vi "PC_Shot_Calculations (DONE).vi"(5 "Table Walls Input":sgl[](array[numeric]), 7 "Player and Puck Input":T1, 8 "Error In":errorcluster) -> (0 "Error Out":errorcluster, 2 "Shot Outputs":cluster{"Bounce":dbl[][], "Straight":dbl[][]})   [LabVIEW 2017]
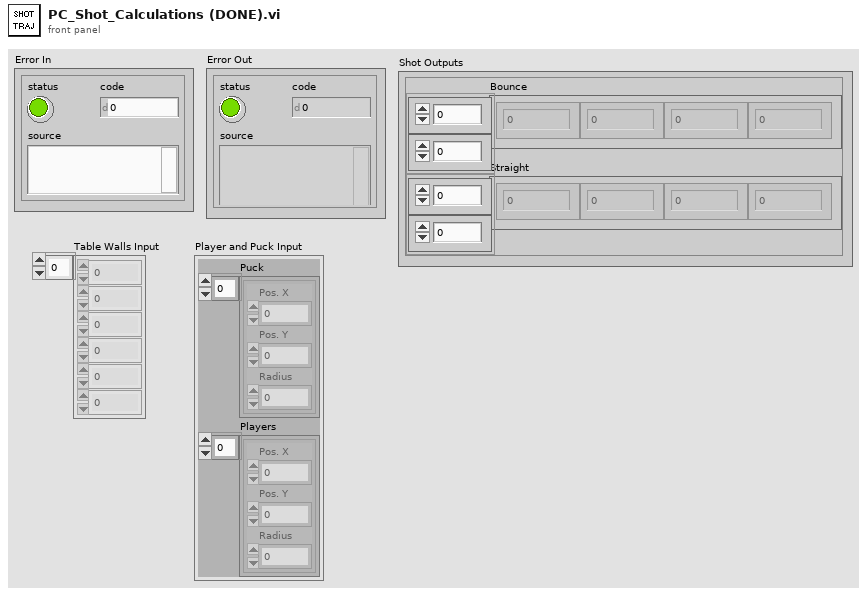
[diagram p1: front panel]
types:
  T1 = cluster{"Puck":cluster{"Pos. X":i32, "Pos. Y":i32, "Radius":i32}[], "Players":cluster{"Pos. X":i32, "Pos. Y":i32, "Radius":i32}[]}
  T2 = cluster{"Pos. X":i32, "Pos. Y":i32, "Radius":i32}[]
  T3 = cluster{"Pos. X":i32, "Pos. Y":i32, "Radius":i32}
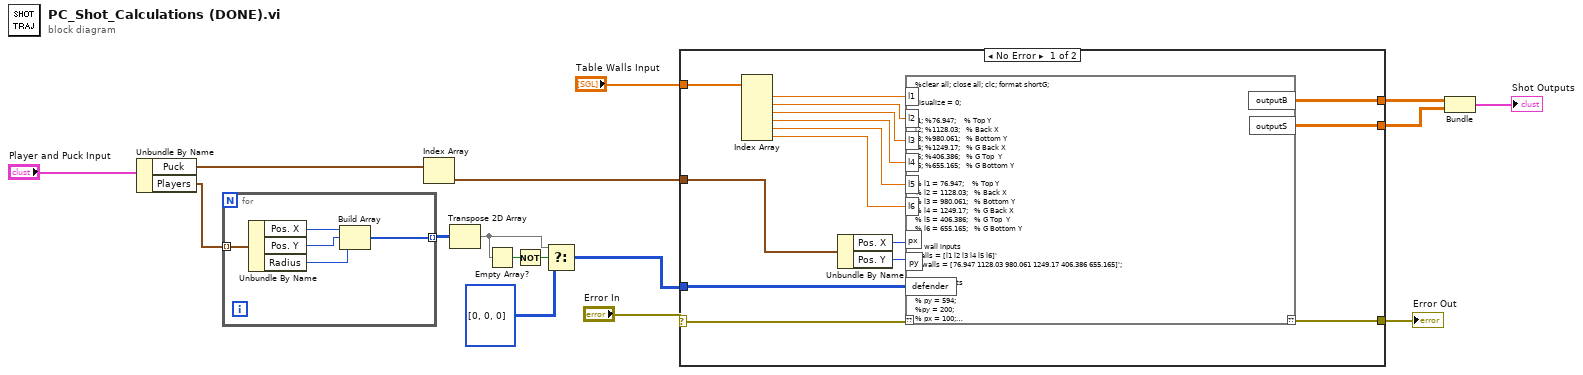
[diagram p0: block diagram]
diagram:
  n1 = Unbundle By Name("Player and Puck Input") -> ("Puck"=w14:T2, "Players"=w10:T2)
  n2 = for {
    tunnel: w10 -> [w21] mode=indexing
    tunnel: [w17] -> w9 mode=indexing
    n3 = Unbundle By Name(w21) -> ("Pos. X"=w20:i32, "Pos. Y"=w19:i32, "Radius"=w18:i32)
    n4 = Build Array(w20, w19, w18) -> (w17:i32[])
  }
  n5 = Index Array(array=w14) -> (element=w11:T3)  [unwired: 1 in]
  n6 = Transpose 2D Array(2D array=w9) -> (transposed array=w6:i32[][])
  n7 = Empty Array?(array=w6) -> (empty?=w8:bool)
  n8 = Not(x=w8) -> (.not. x?=w7:bool)
  n9 = Select(t=w6, s=w7, f=i32[][] [[0], [0], [0]]) -> (s? t:f=w5:i32[][])
  n10 = case shown="No Error" "Error In" {
    selector: "Error In" -> [w35 w37]
    tunnel: [w36 w37] -> w16
    tunnel: [w34 _] -> w3
    tunnel: [w33 _] -> w2
    tunnel: w5 -> [w32 _]
    tunnel: "Table Walls Input" -> [w31 _]
    tunnel: w11 -> [w24 _]
    frame No Error {
      n11 = Index Array(array=w31) -> (element #1=w30:sgl, element #2=w29:sgl, element #3=w28:sgl, element #4=w27:sgl, element #5=w26:sgl, element #6=w25:sgl)  [unwired: 6 in]
      n12 = Unbundle By Name(w24) -> ("Pos. X"=w23:i32, "Pos. Y"=w22:i32)
      n13 = script code="%clear all; close all; clc; format shortG;\n\nvisualize = 0;\n\nl1; %76.947;    % Top Y\nl2; %1128.03;   % Back X\nl3; %980.061;   % Bottom Y\nl4; %1249.17;   % G Back X\nl5; %406.386;   % G Top  Y\nl6; %655.165;   % G Bottom Y\n\n% l1 = 76.947;    % Top Y\n% l2 = 1128.03;   % Back X\n% l3 = 980.061;   % Bottom Y\n% l4 = 1249.17;   % G Back X\n% l5 = 406.386;   % G Top  Y\n% l6 = 655.165;   % G Bottom Y\n\n% wall inputs\nwalls = [l1 l2 l3 l4 l5 l6]'\n%walls = [76.947 1128.03 980.061 1249.17 406.386 655.165]';\n\n% puck inputs\n% px = 359;\n% py = 594;\n%py = 200;\n% px = 100;\n% py = 500;\npx;\npy;\n\n% dx = 800;\n% dy = 500;\n% dr = 80;\n\n% defender inputs blue 1, red 2, yellow 3\n% defender = [844 841 523 847;\n%             411 624  721 856;\n%             38  38   38 38];\n% defender = [0;\n%             0;\n%             0];\n% defender = [600;\n%             200;\n%             dr];\n\ndefender;\n\n% radius of imaginary circle off image for line plotting\nr = 5000;\n\n% min and max angle of theta shots\nminTheta = -72;\nmaxTheta = 72;\n\nif visualize\n    % plot pitch\n    xlim = 1300;\n    ylim = 1049;\n    line([0 walls(2)], [walls(1),walls(1)])      % l1\n    line([walls(2), walls(2)], [walls(1),walls(5)])    % l2\n    pl = line([walls(2), walls(2)], [walls(5),walls(6)]);    % l2\n    pl.Color = 'red';\n    pl.LineStyle = '--';\n    line([walls(2), walls(2)], [walls(6),walls(3)])    % l2\n    line([0 walls(2)], [walls(3),walls(3)])      % l3\n    line([walls(4), walls(4)], [walls(5),walls(6)])    % l4\n    line([walls(2) walls(4)], [walls(5),walls(5)])     % l5\n    line([walls(2) walls(4)], [walls(6),walls(6)])     % l6\n    axis([0 walls(4) walls(1) walls(3)])\n    set(gca,'Ydir','reverse');\n    hold on\n    plot(px,py,'r*')\nend\n\n%% calculate all initial shots\ntheta = minTheta:0.9:maxTheta;\n\n% x,y on imaginary circle\ninit_x = r*cos(theta*pi/180)+px;\ninit_y = r*sin(theta*pi/180)+py;\n\n% calculate line coefficients from puck to imaginary circle\nfor i = 1:length(theta)\n    coeffp_c(i,:) = polyfit([px, init_x(i)], [py, init_y(i)], 1);\nend\ninit_m = coeffp_c(:,1);\ninit_c = coeffp_c(:,2);\n\n% calculate line coefficients from puck to defenders\nfor i = 1:size(defender,2)\n    coeffp_d(i,:) = polyfit([px, defender(1,i)], [py, defender(2,i)], 1);\nend\nd_m = coeffp_d(:,1);\nd_c = coeffp_d(:,2);\n\nif visualize\n    % plot pucks\n    for i = 1:size(defender,2)\n        th = 0:pi/50:2*pi;\n        xunit = defender(3,i) * cos(th) + defender(1,i);\n        yunit = defender(3,i) * sin(th) + defender(2,i);\n        h = plot(xunit, yunit);\n        hold on\n    end\nend\n\n% calculate intersecting triangles between puck and defenders\nxpd = defender(1,:)-px;\nypd = defender(2,:)-py;\npd = sqrt((xpd.^2) + (ypd.^2));\nthd = (asin(defender(3,:)./pd))*180/pi;\nthpd = (acos(xpd./pd))*180/pi;\nfor i = 1:size(defender,2)\n    if ypd(i) > 0\n        thpd(i) = -thpd(i);\n    end\nend\n\n% makes theta NaN if intersecting defenders\nfor j = 1:size(defender,2)\n    for i = 1:length(theta)\n        if ~(theta(i) >= -thpd(j)+thd(j) || theta(i) <= -thpd(j)-thd(j))\n            theta(i) = NaN;\n        end\n    end\nend\n\n% calculate interceptions of l2\n% bellow goal\nxpgb = atan((walls(6)-py)/(walls(2)-px))*180/pi;\nxpl3 = atan((walls(3)-py)/(walls(2)-px))*180/pi;\n\nfor i = 1:length(theta)\n    if ~(theta(i) <= xpgb || theta(i) >= xpl3)\n        theta(i) = NaN;\n    end\nend\n\n% above goal\nxpgt = atan((py-walls(5))/(walls(2)-px))*180/pi;\nxpl1 = atan((py-walls(1))/(walls(2)-px))*180/pi;\n\nfor i = 1:length(theta)\n    if ~(theta(i) <= -xpl1 || theta(i) >= -xpgt)\n        theta(i) = NaN;\n    end\nend\n\n% calculate intersection points between inital shots and walls\nl1_inter = (walls(1) - init_c)./init_m;\nl2_inter = (init_m*walls(2))+init_c;\nl3_inter = (walls(3) - init_c)./init_m;\n\n% eliminate shots behind puck and not in required areas\nl1_inter(l1_inter>=walls(2)) = NaN;\nl1_inter(l1_inter<=px) = NaN;\nl2_inter(l2_inter<=walls(5)) = NaN;\nl2_inter(l2_inter>=walls(6)) = NaN;\nl3_inter(l3_inter>=walls(2)) = NaN;\nl3_inter(l3_inter<=px) = NaN;\n\nfor i = 1:length(l3_inter)\n    %plot([l3_inter(i) walls(2)], [walls(3) yil3l2(i)],'g')\n    %hold on;\nend\n\n% top shot puck collisions\nxil1d = defender(1,:)-l1_inter;\nyil2d = defender(2,:)-walls(1);\nil1d = sqrt((xil1d.^2)+(yil2d.^2));\nrhod = (asin((defender(3,:))./il1d))*180/pi;\nrhoid = (acos(xil1d./il1d))*180/pi;\n\nfor j = 1:size(defender,2)\n    for i = 1:size(l1_inter)\n        if  (-theta(i) <= rhod(i,j)+rhoid(i,j) && -theta(i) >= rhoid(i,j)-rhod(i,j))\n            theta(i) = NaN;\n            l1_inter(i) = NaN;\n            yil1l2(i) = NaN;\n        end\n    end\nend\n\nxid = defender(1,:)-l3_inter;\nyid = walls(3)-defender(2,:);\nid = sqrt((xid.^2)+(yid.^2));\nrhod = (asin((defender(3,:))./id))*180/pi;\nrhoid = (acos(xid./id))*180/pi;\n\nfor j = 1:size(defender,2)\n    for i = 1:size(l3_inter)\n        if  (theta(i) <= rhod(i,j)+rhoid(i,j) && theta(i) >= rhoid(i,j)-rhod(i,j))\n            theta(i) = NaN;\n            l3_inter(i) = NaN;\n            yil3l2(i) = NaN;\n        end\n    end\nend\n\n\n% top bounce\nfor i = 1:length(l1_inter)\n    xil1l2(i) = walls(2)-l1_inter(i);\n    yil1l2(i) = -xil1l2(i)*tan(theta(i)*pi/180)+walls(1);\n    if ~(yil1l2(i) <= walls(5) || yil1l2(i) >= walls(6))\n        if visualize\n            plot([l1_inter(i) walls(2)], [walls(1) yil1l2(i)],'g')\n            hold on\n        end\n    else\n        l1_inter(i) = NaN;\n        theta(i) = NaN;\n        yil1l2(i) = NaN;\n    end\n    \nend\n\n% bottom bounce\nfor i = 1:length(l3_inter)\n    xil3l2(i) = walls(2)-l3_inter(i);\n    yil3l2(i) = walls(3)-(xil3l2(i)*tan(theta(i)*pi/180));\n    if ~(yil3l2(i) <= walls(5) || yil3l2(i) >= walls(6))\n        if visualize\n            plot([l3_inter(i) walls(2)], [walls(3) yil3l2(i)],'g')\n            hold on\n        end\n    else\n        l3_inter(i) = NaN;\n        theta(i) = NaN;\n        yil3l2(i) = NaN;\n    end\nend\n\nfor i = 1:length(l1_inter)\n    if ~isnan(theta(i))\n        if visualize\n            plot([px init_x(i)], [py init_y(i)],'g')\n        end\n    else\n        l1_inter(i) = NaN;\n        l2_inter(i) = NaN;\n        l3_inter(i) = NaN;\n    end\nend\n\nif visualize\n    % plot wall interceptions\n    plot(l1_inter,walls(1),'ro') %l1 intercepts\n    hold on\n    plot(walls(2),l2_inter,'r*') %goal straight intercepts\n    hold on\n    plot(l3_inter,walls(3),'ro') %l3 intercepts\n    hold on\n    plot(walls(2),yil1l2,'bo') %l1 goal intercepts\n    hold on\n    plot(walls(2),yil3l2,'bo') %l2 goal intercepts\n    hold on\nend\n\n% theta, X intercept points wall rebounds, Y intercepts points wall\n% rebounds.\noutputB = NaN(length(theta),3);\noutputS = NaN(length(theta),3);\noutputB(:,1) = theta;\noutputS(:,1) = theta;\n\n% l1 intercept points\nfor i = 1:length(l1_inter)\n    if ~isnan(l1_inter(i))\n        outputB(i,2) = l1_inter(i);\n    end\nend\n\n% l1 goal intercept points\nfor i = 1:length(yil1l2)\n    if ~isnan(yil1l2(i))\n        outputB(i,3) = yil1l2(i);\n    end\nend\n\n% l3 intercept points\nfor i = 1:length(l3_inter)\n    if ~isnan(l3_inter(i))\n        outputB(i,2) = l3_inter(i);\n    end\nend\n\n% l3 goal intercept points\nfor i = 1:length(yil3l2)\n    if ~isnan(yil3l2(i))\n        outputB(i,3) = yil3l2(i);\n    end\nend\n\n% l2 intercept points\nfor i = 1:length(l2_inter)\n    if ~isnan(l2_inter(i))\n        outputS(i,2) = walls(2);\n        outputS(i,3) = l2_inter(i);\n    end\nend\n\noutputB(any(isnan(outputB),2),:) = [];\noutputS(any(isnan(outputS),2),:) = [];\noutputB;\noutputS;"("??"=w35, "l1"=w30, "l2"=w29, "l3"=w28, "l4"=w27, "l5"=w26, "l6"=w25, "px"=w23, "py"=w22, "defender"=w32) -> ("??"=w36:errorcluster, "outputB"=w34:dbl[][], "outputS"=w33:dbl[][])
    }
    frame Error {
    }
  }
  "Error Out" <- w16
  n14 = Bundle(w3, w2) -> (→"Shot Outputs":cluster{dbl[][], dbl[][]})  [unwired: 1 in]
